vi "Create Type Definition.vi"(8 "error in (no error)":errorcluster, 11 "Application in":refnum<vi>) -> (0 "error out":errorcluster, 2 "TypeDef out":refnum<vi>, 3 "Application out":refnum<vi>)   [LabVIEW 2019, in "VI Scripting Tools.lvlib"]
uses:
  VI Scripting Tools.lvlib
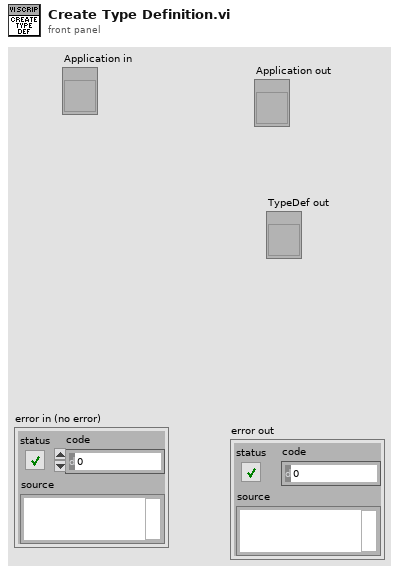
[diagram p1: front panel]
types:
  T1 = enum32{"not a control VI", "control", "typedef", "strict typedef"}
  T2 = enum32{"invalid VI type", "Standard VI", "Control VI", "Global VI", "Polymorphic VI", "Configuration VI", "SubSystem", "Facade VI", "Method VI", "Statechart Diagram VI"}
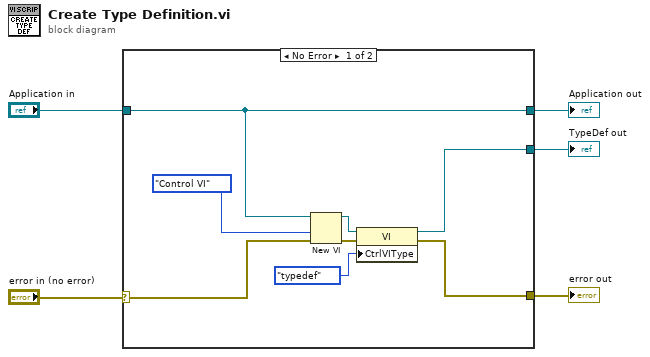
[diagram p0: block diagram]
diagram:
  n1 = case shown="No Error" "error in (no error)" {
    selector: "error in (no error)" -> [w7 w14]
    tunnel: [w13 w14] -> w5
    tunnel: [w12 _] -> w4
    tunnel: "Application in" -> [w6 w15]
    tunnel: [w6 w15] -> w1
    frame No Error {
      n2 = New VI(8:w7, 9:T2."Control VI" ("vi type (standard vi)"), 11:w6) -> (0:w10:errorcluster, 3:w11:refnum<vi>)  [unwired: 4 in]
      n3 = property class="VI"(reference=w11, error in=w10, "CtrlVIType"=T1."typedef" ("Control VI Type")) -> (reference out=w12:refnum<vi>, error out=w13:errorcluster)
    }
    frame Error {
    }
  }
  "error out" <- w5
  "TypeDef out" <- w4
  "Application out" <- w1
